vi "Apply Trim.vi"(8 "Backwards Tuning":T1, 9 "Forward Tuning":T1, 10 "Speed":dbl, 11 "Turn":dbl) -> (3 "Trimmed Turn":dbl)   [LabVIEW 2016]
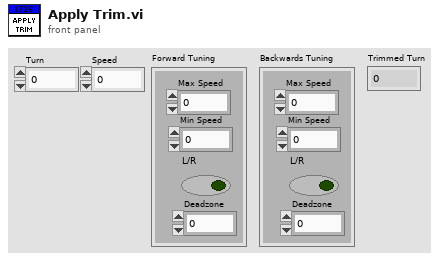
[diagram p1: front panel]
types:
  T1 = cluster{"Max Speed":dbl, "Min Speed":dbl, "L/R":bool, "Deadzone":dbl}
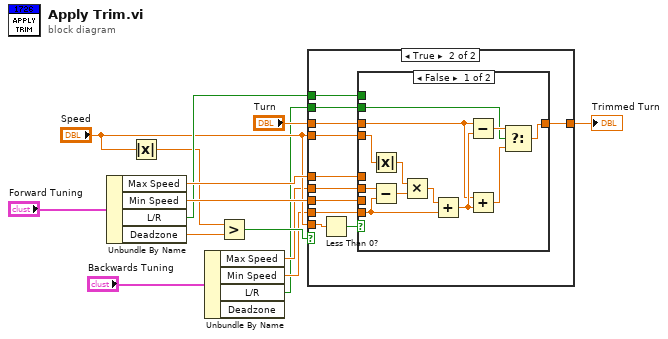
[diagram p0: block diagram]
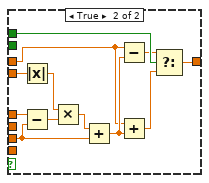
[diagram p3: hidden frame]
diagram:
  n1 = Unbundle By Name("Forward Tuning") -> ("Max Speed"=w13:dbl, "Min Speed"=w12:dbl, "L/R"=w11:bool, "Deadzone"=w9:dbl)
  n2 = Absolute Value(x="Speed") -> (abs(x)=w10:dbl)
  n3 = Unbundle By Name("Backwards Tuning") -> ("Max Speed"=w3:dbl, "Min Speed"=w2:dbl, "L/R"=w1:bool)  [unwired: 1 out]
  n4 = Greater?(x=w10, y=w9) -> (0:w6:bool)
  n5 = case shown="True" w6 {
    tunnel: w13 -> [_ w26]
    tunnel: w12 -> [_ w21]
    tunnel: w11 -> [_ w25]
    tunnel: "Speed" -> [_ w24]
    tunnel: "Turn" -> [w15 w23]
    tunnel: [w15 w22] -> w7
    tunnel: "Speed" -> [_ w20]
    tunnel: w3 -> [_ w18]
    tunnel: w2 -> [_ w17]
    tunnel: w1 -> [_ w16]
    frame False {
    }
    frame True {
      n6 = Less Than 0?(x=w20) -> (x < 0?=w19:bool)
      n7 = case shown="False" w19 {
        tunnel: w26 -> [_ w50]
        tunnel: w25 -> [_ w48]
        tunnel: w24 -> [w30 w39]
        tunnel: w23 -> [w27 w44]
        tunnel: [w32 w43] -> w22
        tunnel: w21 -> [_ w41]
        tunnel: w18 -> [w29 _]
        tunnel: w17 -> [w28 _]
        tunnel: w16 -> [w31 _]
        frame False {
          n8 = Absolute Value(x=w30) -> (abs(x)=w33:dbl)
          n9 = Subtract(x=w29, y=w28) -> (x-y=w38:dbl)
          n10 = Multiply(x=w33, y=w38) -> (x*y=w34:dbl)
          n11 = Add(x=w34, y=w28) -> (x+y=w36:dbl)
          n12 = Subtract(x=w27, y=w36) -> (x-y=w35:dbl)
          n13 = Add(x=w27, y=w36) -> (x+y=w37:dbl)
          n14 = Select(t=w35, s=w31, f=w37) -> (s? t:f=w32:dbl)
        }
        frame True {
          n15 = Absolute Value(x=w39) -> (abs(x)=w40:dbl)
          n16 = Subtract(x=w50, y=w41) -> (x-y=w49:dbl)
          n17 = Multiply(x=w40, y=w49) -> (x*y=w42:dbl)
          n18 = Add(x=w42, y=w41) -> (x+y=w46:dbl)
          n19 = Subtract(x=w44, y=w46) -> (x-y=w45:dbl)
          n20 = Add(x=w44, y=w46) -> (x+y=w47:dbl)
          n21 = Select(t=w45, s=w48, f=w47) -> (s? t:f=w43:dbl)
        }
      }
    }
  }
  "Trimmed Turn" <- w7
